vi "TakeFromReference.vi"(8 "error in (no error)":errorcluster, 11 "Refnum in":refnum<k34>) -> (0 "error out":errorcluster, 2 "Referencia":T1[][](array[typedef]), 3 "Refnum out":refnum<k34>)   [LabVIEW 2021]
uses:
  Typedefs/Detected peaks.ctl
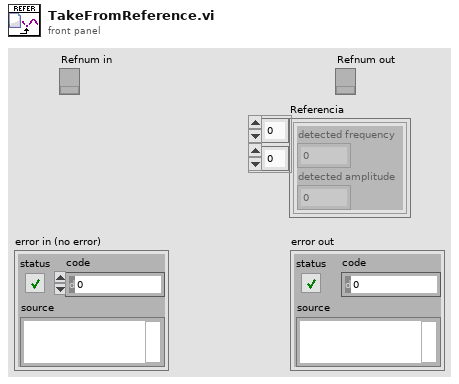
[diagram p1: front panel]
types:
  T1 = typedef "Detected peaks.ctl" = cluster{"detected frequency":dbl, "detected amplitude":dbl}
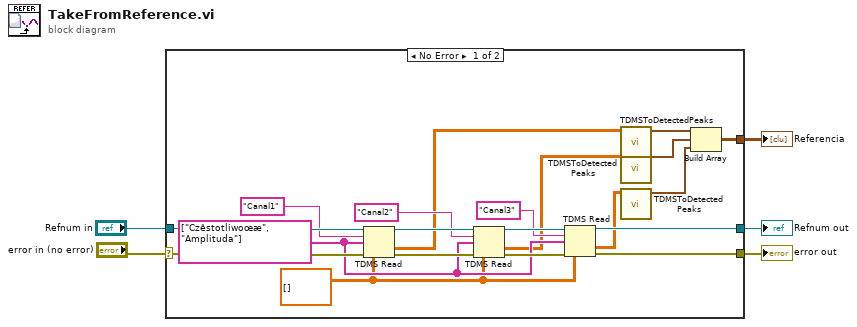
[diagram p0: block diagram]
diagram:
  n1 = case shown="No Error" "error in (no error)" {
    selector: "error in (no error)" -> [w25 w26]
    tunnel: [w17 w26] -> w4
    tunnel: [w18 w27] -> w3
    tunnel: "Refnum in" -> [w24 w27]
    tunnel: [w10 _] -> w1
    frame No Error {
      w9 = dbl[][] [] ("Array")
      w16 = string[] ["Czêstotliwoœæ", "Amplituda"] ("channel name(s) in (Untitled)")
      n2 = TDMS Read(0:w24, 5:"Canal1" ("group name in (Untitled)"), 7:w16, 11:w25, 12:w9) -> (4:w22:refnum<k34>, 10:w8:dbl[][], 15:w21:errorcluster)  [unwired: 3 in, 3 out]
      n3 = TDMS Read(0:w22, 5:"Canal2" ("group name in (Untitled)"), 7:w16, 11:w21, 12:w9) -> (4:w20:refnum<k34>, 10:w7:dbl[][], 15:w19:errorcluster)  [unwired: 3 in, 3 out]
      n4 = TDMS Read(0:w20, 5:"Canal3" ("group name in (Untitled)"), 7:w16, 11:w19, 12:w9) -> (4:w18:refnum<k34>, 10:w6:dbl[][], 15:w17:errorcluster)  [unwired: 3 in, 3 out]
      n5 = call "TDMSToDetectedPeaks.vi"("Array"=w8) -> ("Detected peaks"=w13:T1[])  [unwired: 10 in]
      n6 = call "TDMSToDetectedPeaks.vi"("Array"=w7) -> ("Detected peaks"=w12:T1[])  [unwired: 10 in]
      n7 = call "TDMSToDetectedPeaks.vi"("Array"=w6) -> ("Detected peaks"=w11:T1[])  [unwired: 10 in]
      n8 = Build Array(w13, w12, w11) -> (w10:T1[][])
    }
    frame Error {
    }
  }
  "error out" <- w4
  "Refnum out" <- w3
  "Referencia" <- w1
